vi "HiFiveUnmatched_Main.vi"() -> ()   [LabVIEW 2020]
uses:
  HiFiveUnmatched_PowerLineId.ctl
  <vilib>/DAQmx/read.llb/DAQmx Read (Analog 1D Wfm NChan NSamp).vi
  <extravilib>/ChannelInstances/Stream-a[.](wfm(dbl))/EndpointRead.vi
  <extravilib>/ChannelInstances/Stream-a[.](wfm(dbl))/Endpoint.vi
  <extravilib>/ChannelInstances/Stream-a[.](wfm(dbl))/Instantiate.vi
  <extravilib>/ChannelInstances/Stream-a[.](wfm(dbl))/)Channel.vi
  <resource>/ChannelSupport/_ChannelSupport/WaitIfNeeded.vi
  <vilib>/DAQmx/miscellaneous.llb/DAQmx Fill In Error Info.vi
  <extravilib>/ChannelInstances/Stream-a[.](wfm(dbl)).lvlib
panel:
  out "Power Monitor":waveform(dbl)[](graph)
  in  "File Update Time":u32=900
  in  "Experiment Name":string
  in  "Log Directory Path":path
  in  "STOP":bool
  in  "Rate Selection":enum32{"Auto", "Manual"}(radio)=enum."Manual"
  in  "Sampling Rate [Hz]":dbl(knob)=50000.0 min=1000.0 max=2000000.0 step=1000.0 scale=1000.0..2000000.0 scale format="%#.1p"
  in  "START":bool
  in  "Enable Channel\nDDR_VPP":bool=TRUE
  in  "Enable Channel\nPCIEVPH":bool=TRUE
  in  "Enable Channel\nIO":bool=TRUE
  in  "Channel\nDDR_VPP":tag="PXIe-4309/ai30"
  in  "Channel\nPCIEVPH":tag="PXIe-4309/ai26"
  in  "Channel\nIO":tag="PXIe-4309/ai31"
  in  "Enable Channel\nDDR_PLL":bool=TRUE
  in  "Enable Channel\nPCIEVP":bool=TRUE
  in  "Enable Channel\nDDR_SOC":bool=TRUE
  in  "Channel\nDDR_PLL":tag="PXIe-4309/ai29"
  in  "Channel\nPCIEVP":tag="PXIe-4309/ai4"
  in  "Channel\nDDR_SOC":tag="PXIe-4309/ai25"
  in  "Enable Channel\nDDR_MEM":bool=TRUE
  in  "Enable Channel\nPLL":bool=TRUE
  in  "Enable Channel\nCORE":bool=TRUE
  in  "Channel\nDDR_MEM":tag="PXIe-4309/ai27"
  in  "Channel\nPLL":tag="PXIe-4309/ai24"
  in  "Channel\nCORE":tag="PXIe-4309/ai28"
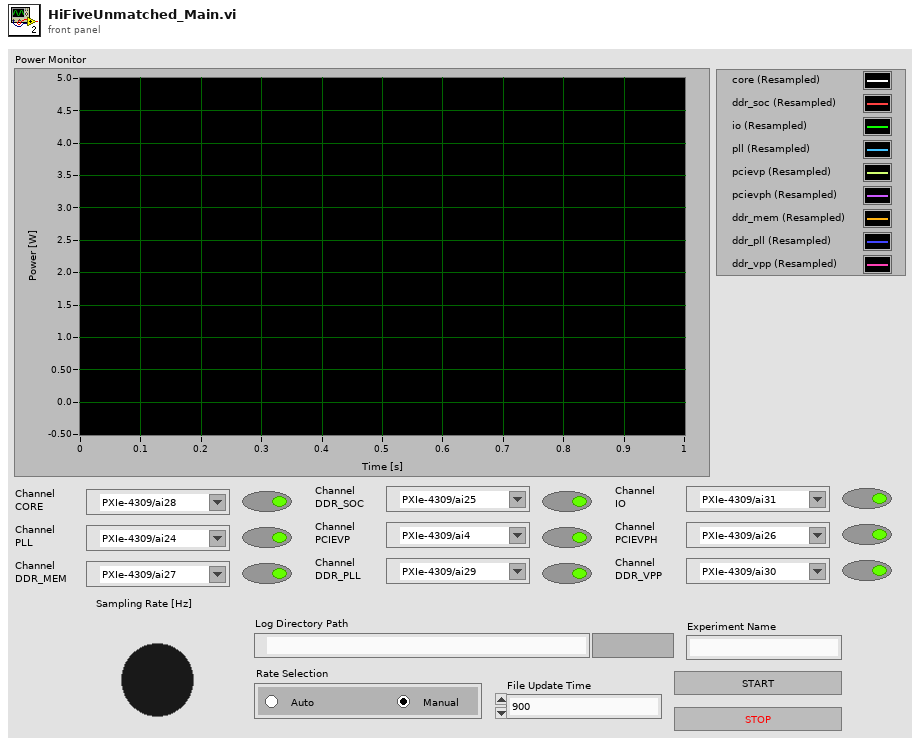
[diagram p1: front panel]
types:
  T1 = enum16{"big-endian, network order", "native, host order", "little-endian"}
  T2 = enum16{"open", "open or create", "create or replace", "create", "open (read-only)"}
  T3 = typedef "HiFiveUnmatched_PowerLineId.ctl" = enum8{"CORE", "DDR_SOC", "IO", "PLL", "PCIEVP", "PCIEVPH", "DDR_MEM", "DDR_PLL", "DDR_VPP"}
  T4 = typedef "HiFiveUnmatched_PowerLineCfg.ctl" = cluster{"Name":string, "Shunt [Ohm]":dbl, "Min Current [A]":dbl, "Max Current [A]":dbl, "Voltage [V]":dbl, "Physical Channel":tag, "Enable":bool}
  T5 = typedef "Stream-a[.](wfm(dbl)).lvlib/)Channel.ctl" = refnum<queue>
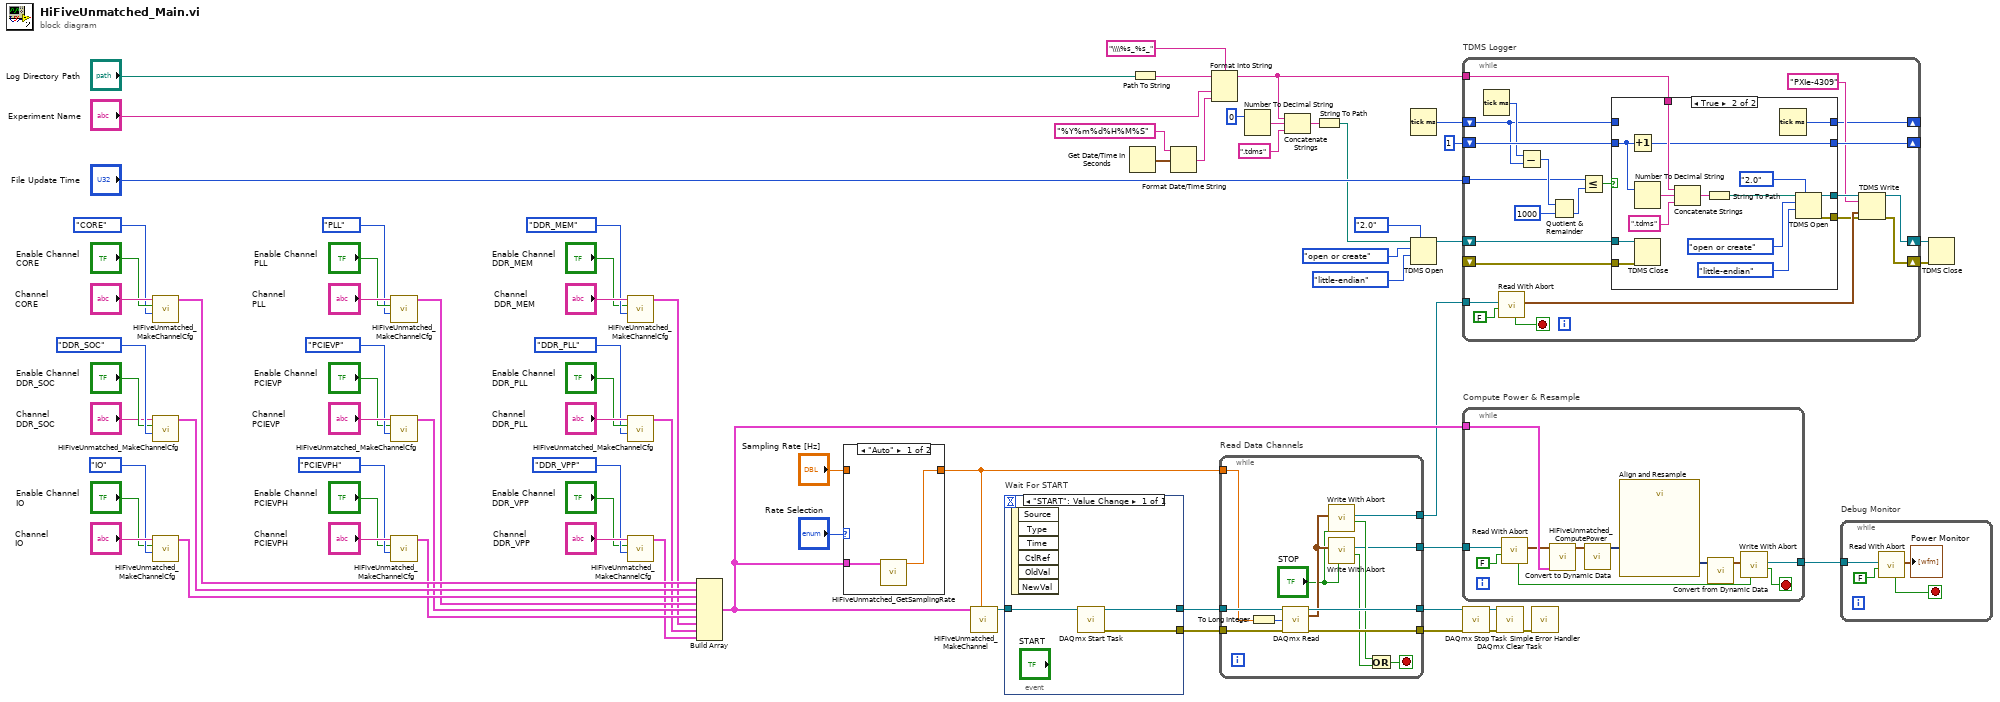
[diagram p0: block diagram]
diagram:
  n1 = call "HiFiveUnmatched_MakeChannelCfg.vi"("Power Line Identifier"=HiFiveUnmatched_PowerLineId."CORE", "Enable"="Enable Channel\nCORE", "Physical Channel"="Channel\nCORE") -> ("Configuration"=w46:T4)  [unwired: 8 in]
  n2 = call "HiFiveUnmatched_MakeChannelCfg.vi"("Power Line Identifier"=HiFiveUnmatched_PowerLineId."DDR_SOC", "Enable"="Enable Channel\nDDR_SOC", "Physical Channel"="Channel\nDDR_SOC") -> ("Configuration"=w45:T4)  [unwired: 8 in]
  n3 = call "HiFiveUnmatched_MakeChannelCfg.vi"("Power Line Identifier"=HiFiveUnmatched_PowerLineId."IO", "Enable"="Enable Channel\nIO", "Physical Channel"="Channel\nIO") -> ("Configuration"=w44:T4)  [unwired: 8 in]
  n4 = call "HiFiveUnmatched_MakeChannelCfg.vi"("Power Line Identifier"=HiFiveUnmatched_PowerLineId."PLL", "Enable"="Enable Channel\nPLL", "Physical Channel"="Channel\nPLL") -> ("Configuration"=w43:T4)  [unwired: 8 in]
  n5 = call "HiFiveUnmatched_MakeChannelCfg.vi"("Power Line Identifier"=HiFiveUnmatched_PowerLineId."PCIEVP", "Enable"="Enable Channel\nPCIEVP", "Physical Channel"="Channel\nPCIEVP") -> ("Configuration"=w42:T4)  [unwired: 8 in]
  n6 = call "HiFiveUnmatched_MakeChannelCfg.vi"("Power Line Identifier"=HiFiveUnmatched_PowerLineId."PCIEVPH", "Enable"="Enable Channel\nPCIEVPH", "Physical Channel"="Channel\nPCIEVPH") -> ("Configuration"=w41:T4)  [unwired: 8 in]
  n7 = call "HiFiveUnmatched_MakeChannelCfg.vi"("Power Line Identifier"=HiFiveUnmatched_PowerLineId."DDR_MEM", "Enable"="Enable Channel\nDDR_MEM", "Physical Channel"="Channel\nDDR_MEM") -> ("Configuration"=w40:T4)  [unwired: 8 in]
  n8 = call "HiFiveUnmatched_MakeChannelCfg.vi"("Power Line Identifier"=HiFiveUnmatched_PowerLineId."DDR_PLL", "Enable"="Enable Channel\nDDR_PLL", "Physical Channel"="Channel\nDDR_PLL") -> ("Configuration"=w39:T4)  [unwired: 8 in]
  n9 = call "HiFiveUnmatched_MakeChannelCfg.vi"("Power Line Identifier"=HiFiveUnmatched_PowerLineId."DDR_VPP", "Enable"="Enable Channel\nDDR_VPP", "Physical Channel"="Channel\nDDR_VPP") -> ("Configuration"=w38:T4)  [unwired: 8 in]
  n10 = Build Array(w46, w45, w44, w43, w42, w41, w40, w39, w38) -> (w28:T4[])
  n11 = case shown="\"Auto\"" "Rate Selection" {
    tunnel: w28 -> [w75 _]
    tunnel: [w74 w76] -> w27
    tunnel: "Sampling Rate [Hz]" -> [_ w76]
    frame "Auto" {
      n12 = call "HiFiveUnmatched_GetSamplingRate.vi"("Channel Configuration"=w75) -> ("Sampling Rate"=w74:dbl)  [unwired: 10 in]
    }
    frame "Manual" {
    }
  }
  n13 = call "HiFiveUnmatched_MakeChannel.vi"("Sampling Rate [Hz]"=w27, "Power Line Configurations"=w28) -> ("Output Task"=w17:refnum<k21>)  [unwired: 8 in, 1 out]
  n14 = event "Wait For START" shown="[0] \"START\": Value Change" {
    selector: _ -> [_]
    dyn-events: _ -> [_]
    timeout: _ -> [_]
    tunnel: [w79] -> w35
    tunnel: [w78] -> w34
    tunnel: w17 -> [w77]
    event "START": Value Change {
      n15 = event-data() -> ()  [unwired: 1 in, 6 out]
      n16 = call <vilib>:"DAQmx Start Task.vi"("task/channels in"=w77) -> ("task out"=w79:refnum<k21>, "error out"=w78:errorcluster)  [unwired: 13 in]
    }
  }
  n17 = Get Date/Time In Seconds() -> (seconds since 1Jan1904=w21:timestamp)
  n18 = Path To String(path="Log Directory Path") -> (string=w23:string)
  n19 = Format Date/Time String(time format string (%c)="%Y%m%d%H%M%S", seconds (now)=w21) -> (date/time string=w19:string)  [unwired: 1 in]
  n20 = Format Into String(format string="\\\\%s_%s_", initial string=w23, "Experiment Name", w19) -> (resulting string=w15:string)  [unwired: 1 in, 1 out]
  n21 = while "Read Data Channels" {
    tunnel: w27 -> [w87]
    tunnel: w35 -> [w92]
    tunnel: w34 -> [w91]
    tunnel: [w90] -> w30
    tunnel: [w89] -> w29
    tunnel: [w82] -> w5
    tunnel: [w81] -> w4
    stop <- w85 stop-if-true
    n22 = To Long Integer(number=w87) -> (32bit integer=w88:i32)
    n23 = call-poly <vilib>:"DAQmx Read.vi"("task/channels in"=w92, "number of samples per channel"=w88, "error in"=w91) -> ("task out"=w90:refnum<k21>, "data"=w86:waveform(dbl)[], "error out"=w89:errorcluster)  [unwired: 10 in]
    n24 = call <extravilib>:"Write With Abort.vi"("abort"="STOP", "element"=w86) -> ("aborted?"=w83:bool, "channel"=w81:T5)  [unwired: 6 in, 2 out]
    n25 = call <extravilib>:"Write With Abort.vi"("abort"="STOP", "element"=w86) -> ("aborted?"=w84:bool, "channel"=w82:T5)  [unwired: 6 in, 2 out]
    n26 = Or(x=w83, y=w84) -> (x .or. y?=w85:bool)
  }
  n27 = Number To Decimal String(number=0) -> (decimal integer string=w16:string)  [unwired: 1 in]
  n28 = Concatenate Strings(w15, w16, ".tdms" ("string")) -> (w13:string)
  n29 = String To Path(string=w13) -> (path=w9:path)
  n30 = Tick Count (ms)() -> (millisecond timer value=w7:u32)
  n31 = TDMS Open(7:enum16{"1.0", "2.0"}."2.0" ("file format version (2.0)"), 9:T1."little-endian" ("byte order (2:little-endian)"), 10:T2."open or create" ("operation (0:open)"), 11:w9) -> (3:w8:refnum<k34>)  [unwired: 3 in, 1 out]
  n32 = while "TDMS Logger" {
    tunnel: w4 -> [w114]
    tunnel: "File Update Time" -> [w99]
    shift-right: [w109] -> w3
    shift-left: w8 -> [w105]
    shift-right: [w111] -> _
    shift-left: 1 -> [w108]
    tunnel: w15 -> [w106]
    shift-right: [w104] -> _
    shift-left: w7 -> [w102]
    shift-right: [w94] -> w2
    shift-left: _ -> [w93]
    stop <- w113 stop-if-true
    n33 = Tick Count (ms)() -> (millisecond timer value=w103:u32)
    n34 = call <extravilib>:"Read With Abort.vi"("abort"=FALSE ("abort (F)"), "channel"=w114) -> ("element"=w112:waveform(dbl)[], "aborted?"=w113:bool)  [unwired: 4 in, 4 out]
    n35 = Subtract(x=w103, y=w102) -> (x-y=w101:u32)
    n36 = Quotient & Remainder(x=w101, y=u32 1000) -> (floor(x/y)=w98:u32)  [unwired: 1 out]
    n37 = Less Or Equal?(x=w99, y=w98) -> (x <= y?=w97:bool)
    n38 = case shown="True" w97 {
      tunnel: w106 -> [_ w130]
      tunnel: w108 -> [w118 w122]
      tunnel: [w118 w123] -> w111
      tunnel: [w117 w128] -> w110
      tunnel: w105 -> [w117 w127]
      tunnel: [w116 w121] -> w104
      tunnel: w102 -> [w116 _]
      tunnel: [w115 w120] -> w95
      tunnel: w93 -> [w115 w119]
      frame False {
      }
      frame True {
        n39 = Increment(x=w122) -> (x+1=w123:i32)
        n40 = Number To Decimal String(number=w122) -> (decimal integer string=w129:string)  [unwired: 1 in]
        n41 = TDMS Close(8:w119, 11:w127) -> ()  [unwired: 2 out]
        n42 = Concatenate Strings(w130, w129, ".tdms" ("string")) -> (w125:string)
        n43 = String To Path(string=w125) -> (path=w124:path)
        n44 = Tick Count (ms)() -> (millisecond timer value=w121:u32)
        n45 = TDMS Open(7:enum16{"1.0", "2.0"}."2.0" ("file format version (2.0)"), 9:T1."little-endian" ("byte order (2:little-endian)"), 10:T2."open or create" ("operation (0:open)"), 11:w124) -> (0:w120:errorcluster, 3:w128:refnum<k34>)  [unwired: 3 in]
      }
    }
    n46 = TDMS Write(0:w110, 5:"PXIe-4309" ("group name in (Untitled)"), 9:w112, 11:w95) -> (4:w109:refnum<k34>, 15:w94:errorcluster)  [unwired: 2 in, 2 out]
  }
  n47 = while "Compute Power & Resample" {
    tunnel: w5 -> [w144]
    tunnel: w28 -> [w143]
    tunnel: [w134] -> w1
    stop <- w139 stop-if-true
    n48 = call <extravilib>:"Read With Abort.vi"("abort"=FALSE ("abort (F)"), "channel"=w144) -> ("element"=w141:waveform(dbl)[], "aborted?"=w140:bool)  [unwired: 4 in, 4 out]
    n49 = call "HiFiveUnmatched_ComputePower.vi"("Configurations"=w143, "Current Waveforms"=w141) -> ("Power"=w138:waveform(dbl)[])  [unwired: 9 in]
    n50 = call "Convert to Dynamic Data"("Array of Waveforms"=w138) -> ("Dynamic Data Type"=w137:dynamicdata)  [unwired: 3 in]
    n51 = call "Align and Resample"("Signals"=w137) -> ("Resampled Signals"=w136:dynamicdata)  [unwired: 8 in, 2 out]
    n52 = call "Convert from Dynamic Data"("Dynamic Data Type"=w136) -> ("Array of Waveform"=w135:waveform(dbl)[])  [unwired: 3 in]
    n53 = call <extravilib>:"Write With Abort.vi"("abort"=w140, "element"=w135) -> ("aborted?"=w139:bool, "channel"=w134:T5)  [unwired: 6 in, 2 out]
  }
  n54 = call <vilib>:"DAQmx Stop Task.vi"("task/channels in"=w30, "error in"=w29) -> ("task out"=w31:refnum<k21>, "error out"=w33:errorcluster)  [unwired: 12 in]
  n55 = call <vilib>:"DAQmx Clear Task.vi"("task in"=w31, "error in"=w33) -> ("error out"=w32:errorcluster)  [unwired: 13 in]
  n56 = call <vilib>:"Simple Error Handler.vi"("error in (no error)"=w32) -> ()  [unwired: 4 in, 5 out]
  n57 = while "Debug Monitor" {
    tunnel: w1 -> [w148]
    stop <- w147 stop-if-true
    n58 = call <extravilib>:"Read With Abort.vi"("abort"=FALSE ("abort (F)"), "channel"=w148) -> ("element"=→"Power Monitor":waveform(dbl)[], "aborted?"=w147:bool)  [unwired: 4 in, 4 out]
  }
  n59 = TDMS Close(8:w2, 11:w3) -> ()  [unwired: 2 out]
